vi "SubVi-结果计算-从-已知xyk求b.vi"(10 "斜率":dbl, 11 "XY In":dbl[](array[numeric])) -> (3 "解决 Out":dbl)   [LabVIEW 2015]
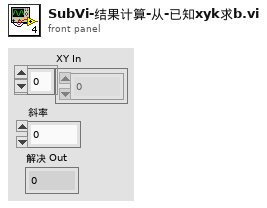
[diagram p1: front panel]
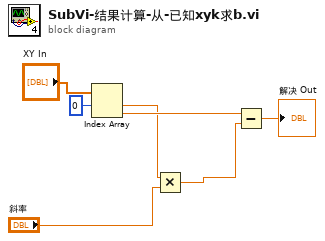
[diagram p0: block diagram]
diagram:
  n1 = Index Array(array="XY In", index #1=0 ("索引")) -> (element #1=w4:dbl, element #2=w5:dbl)  [unwired: 1 in]
  n2 = Multiply(x=w4, y="斜率") -> (x*y=w2:dbl)
  n3 = Subtract(x=w5, y=w2) -> (x-y=→"解决 Out":dbl)
